vi "Slice Engine.vi"(8 "error in (no error)":errorcluster, 11 "System Parameters":T1={"Vibratome"={"Z Bottom [mm]"=0.0, "Pre Cut Dwell [s]"=1.0, "Blade Frequency [RPM]"=3000, "Slice Speed [mm/s]"=1.0, "Post Cut Dwell [s]"=1.0, "Ramp Time [s]"=0.5, "Start X [mm]"=80.5, "Start Y [mm]"=72.0, "Slice Length [mm]"=25.0, "Slice Axis"=enum."X Axis", "Controller VISA Ref"="COM3"}, "Table Stages"={"X Stage"={"Position"=0.0, "Is.Enabled?"=FALSE, "Is.Connected?"=FALSE, "Device SN"="45875688", "AccelerationMaximum"=50.0, "VelocityMaximum"=50.0, "Acceleration"=20.0, "Velocity"=20.0, "waitTimeout (ms)"=1000000, "Model"=enum."Thorlabs LTS", "Is.Homed?"=FALSE}, "Y Stage"={"Position"=0.0, "Is.Enabled?"=FALSE, "Is.Connected?"=FALSE, "Device SN"="45875512", "AccelerationMaximum"=50.0, "VelocityMaximum"=50.0, "Acceleration"=20.0, "Velocity"=20.0, "waitTimeout (ms)"=1000000, "Model"=enum."Thorlabs LTS", "Is.Homed?"=FALSE}, "Z Stage"={"Position"=0.0, "Is.Enabled?"=FALSE, "Is.Connected?"=FALSE, "Device SN"="49872414", "AccelerationMaximum"=50.0, "VelocityMaximum"=50.0, "Acceleration"=20.0, "Velocity"=20.0, "waitTimeout (ms)"=100000, "Model"=enum."Thorlabs MLJ", "Is.Homed?"=FALSE}}}) -> (0 "error out":errorcluster)   [LabVIEW 2017]
uses:
  Controls/System Parameters.ctl
  Hardware/Table Stage/Controls/Translation Stage Cluster.ctl
  Controls/Translation Stage Types.ctl
  Controls/FGV Actions.ctl
  Controls/Queue Manager Actions.ctl
  Controls/QueueNames.ctl
  Hardware/Table Stage/Controls/Motion Translation Module Control.ctl
  Controls/Set Get Controls.ctl
  Controls/Thorlabs Acq Status.ctl
panel:
  in  "Slice thickness  (mm)":dbl=150.0
  in  "Running":bool
  in  "Last Slice?":bool
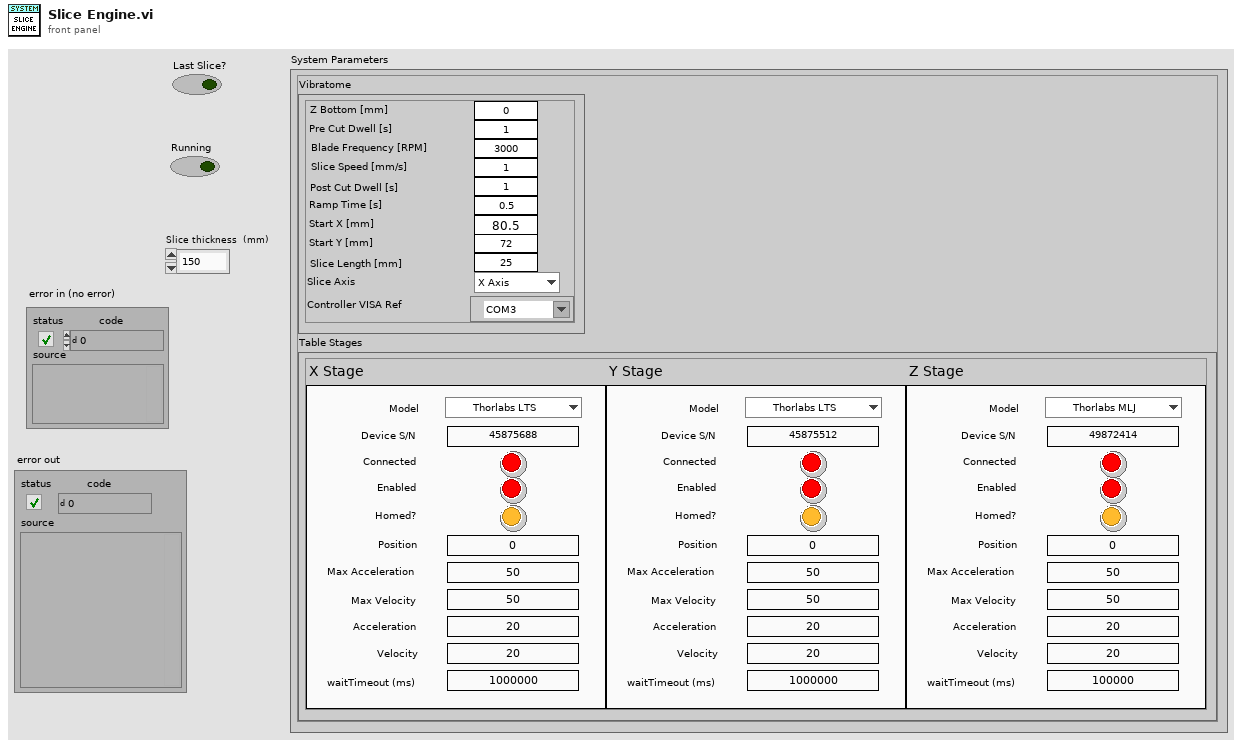
[diagram p1: front panel]
types:
  T1 = typedef "System Parameters.ctl" = cluster{"Vibratome":cluster{"Z Bottom [mm]":dbl, "Pre Cut Dwell [s]":dbl, "Blade Frequency [RPM]":u16, "Slice Speed [mm/s]":dbl, "Post Cut Dwell [s]":dbl, "Ramp Time [s]":dbl, "Start X [mm]":dbl, "Start Y [mm]":dbl, "Slice Length [mm]":dbl, "Slice Axis":enum16{"X Axis", "Y Axis", "Z Axis"}, "Controller VISA Ref":refnum<visa-resource-name>}, "Table Stages":cluster{"X Stage":T2, "Y Stage":T2, "Z Stage":T2}}
  T2 = typedef "Translation Stage Cluster.ctl" = cluster{"Position":dbl, "Is.Enabled?":bool, "Is.Connected?":bool, "Device SN":string, "AccelerationMaximum":dbl, "VelocityMaximum":dbl, "Acceleration":dbl, "Velocity":dbl, "waitTimeout (ms)":i32, "Model":T3, "Is.Homed?":bool}
  T3 = typedef "Translation Stage Types.ctl" = enum16{"None", "Thorlabs LTS", "Thorlabs MLJ"}
  T4 = typedef "FGV Actions.ctl" = enum16{"Init", "Set", "Get", "Clear"}
  T5 = typedef "QueueNames.ctl" = enum16{"Main GUI", "Main Scan Processor", "Main Display", "Main Table Stage GUI", "Main Table Stage Proc.", "Scan Engine", "Vibratome GUI", "Vibratome Processor", "Slice Engine"}
  T6 = typedef "Queue Manager Actions.ctl" = enum16{"Init", "Enqueue", "Enqueue All", "Preview Queue", "Dequeue", "Get Status", "Flush Queue", "Flush All Queues", "Release All Queues", "Release Queue", "Enqueue at Opposite End"}
  T7 = typedef "Set Get Controls.ctl" = enum16{"Set", "Get"}
  T8 = typedef "Motion Translation Module Control.ctl" = enum16{"Init", "Home", "Status", "Velocity/Accel", "Position", "Jog", "Stop", "Uninit", "Enable", "Disable"}
  T9 = enum16{"Set Configuration", "Get Configuration", "Enable Motor", "Disable Motor", "Get Status", "Open Session", "Close Session", "Set Limits", "Get Limits"}
  T10 = cluster{"Source for Velocity":enum16{"Interface", "Voltage (AI)", "PWM (AI)", "Current Target (AI)", "Current Target w/ Preset (AI)"}, "Mode":enum16{"Continuous", "Stepper Motor", "Analog Position Ctrl", "Encoder"}, "Target Velocity [RPM]":i16}
  T11 = typedef "Thorlabs Acq Status.ctl" = enum16{"Idle", "Image", "Translate"}
  T12 = typedef "MessagePacket.ctl" = cluster{"Message":string, "Parameter":variant}
  T13 = cluster{"X Stage":T2, "Y Stage":T2, "Z Stage":T2}
  T14 = cluster{"Z Bottom [mm]":dbl, "Pre Cut Dwell [s]":dbl, "Blade Frequency [RPM]":u16, "Slice Speed [mm/s]":dbl, "Post Cut Dwell [s]":dbl, "Ramp Time [s]":dbl, "Start X [mm]":dbl, "Start Y [mm]":dbl, "Slice Length [mm]":dbl, "Slice Axis":enum16{"X Axis", "Y Axis", "Z Axis"}, "Controller VISA Ref":refnum<visa-resource-name>}
  T15 = enum16{"Left Button", "Center Button", "Right Button", "Window Close"}
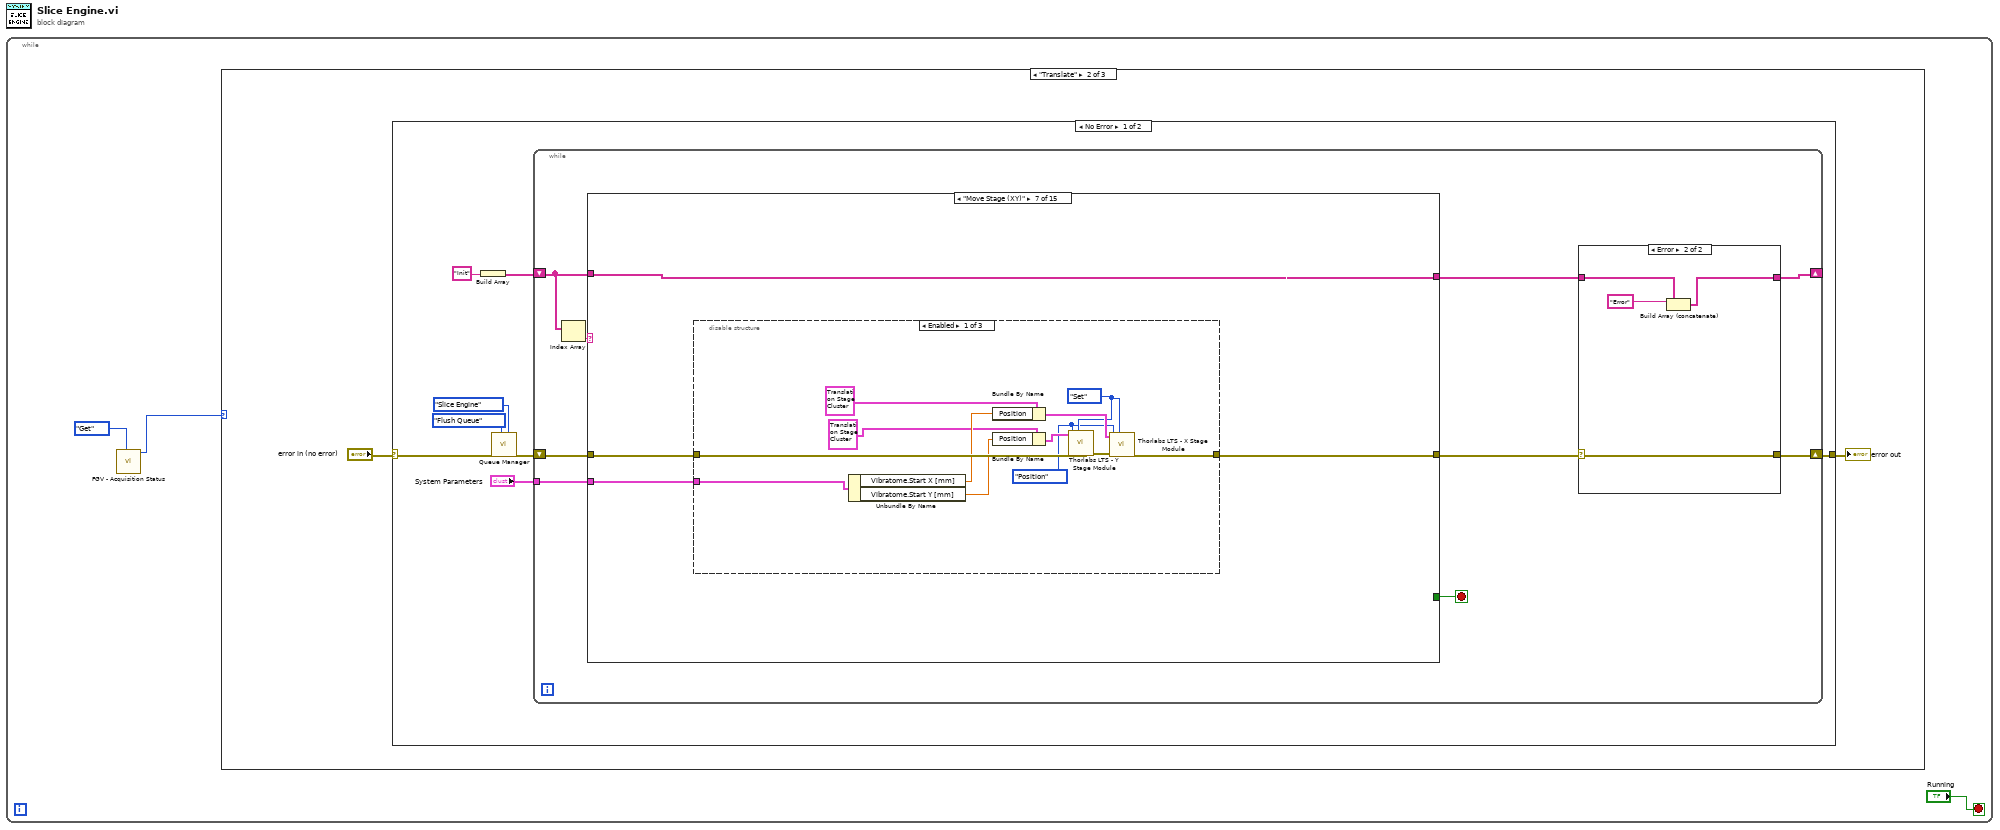
[diagram p0: block diagram]
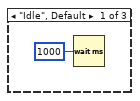
[diagram p2: hidden frame]
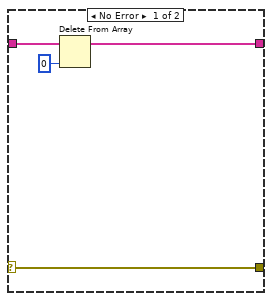
[diagram p3: hidden frame]
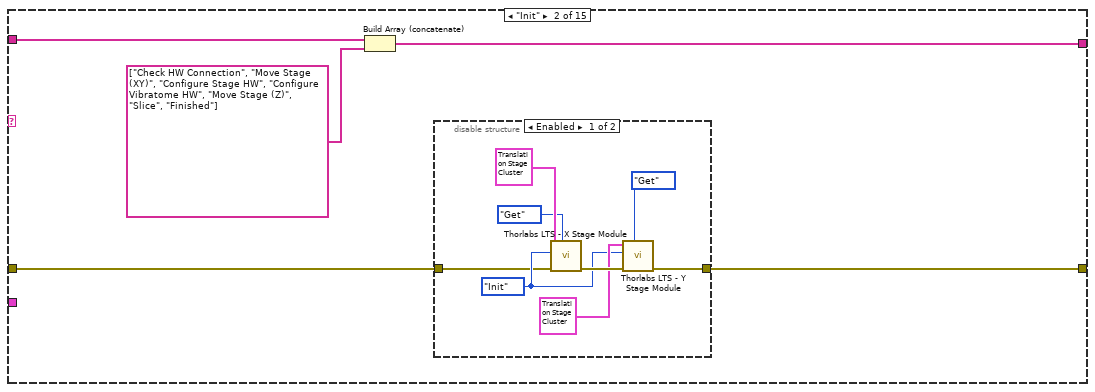
[diagram p5: hidden frame]
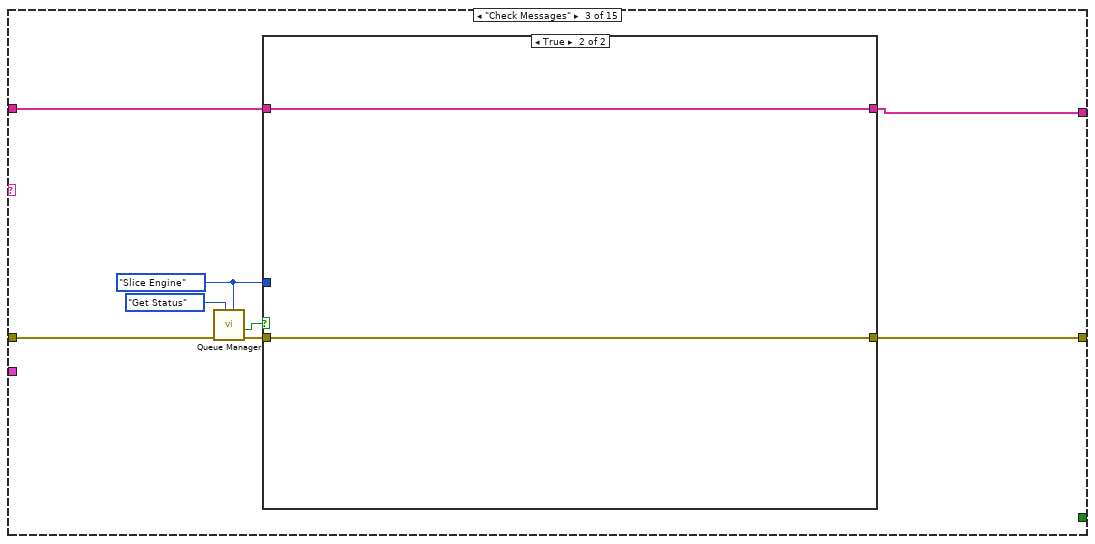
[diagram p7: hidden frame]
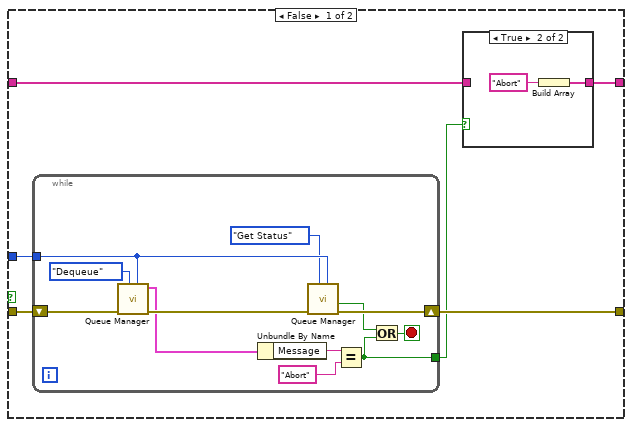
[diagram p8: hidden frame]
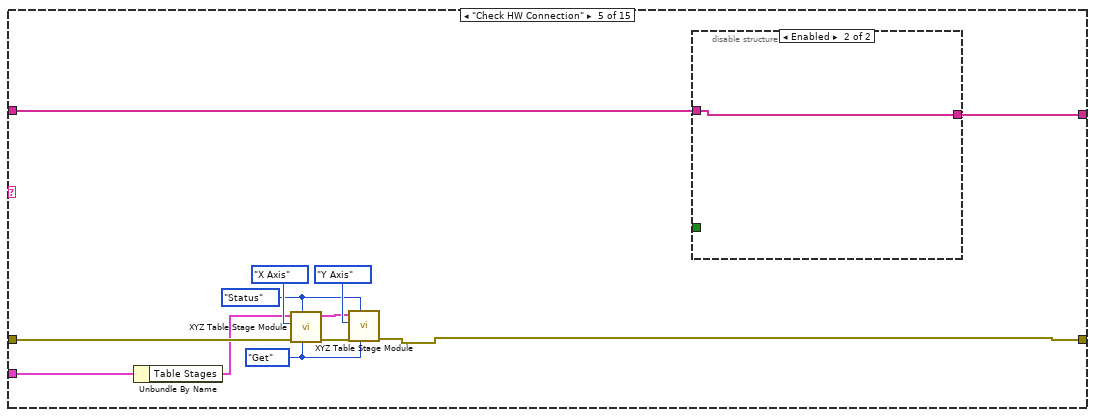
[diagram p11: hidden frame]
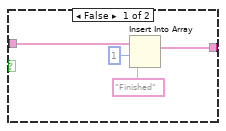
[diagram p13: hidden frame]
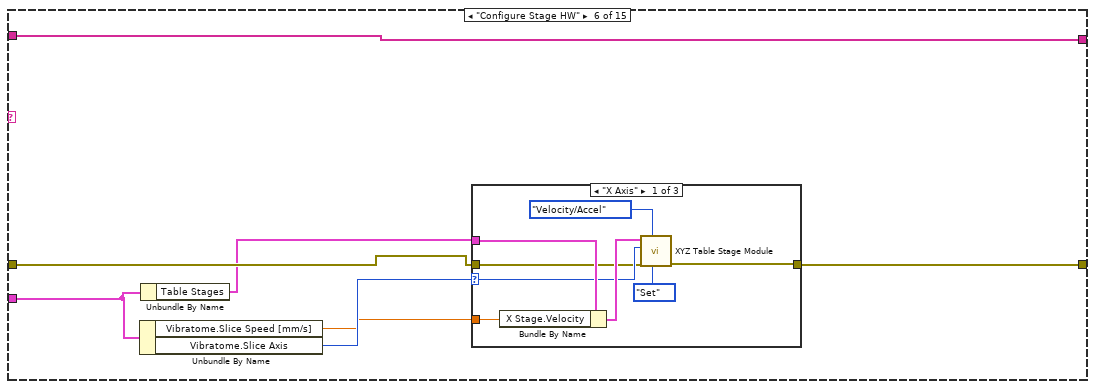
[diagram p14: hidden frame]
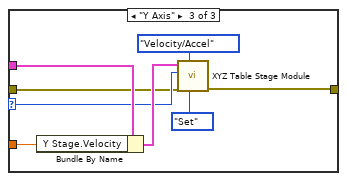
[diagram p16: hidden frame]
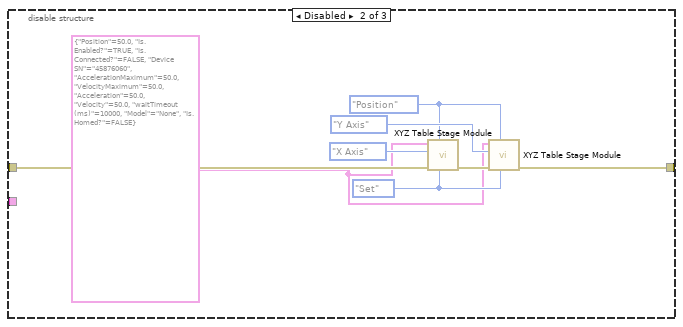
[diagram p17: hidden frame]
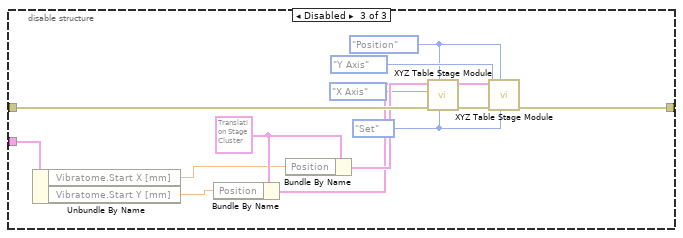
[diagram p18: hidden frame]
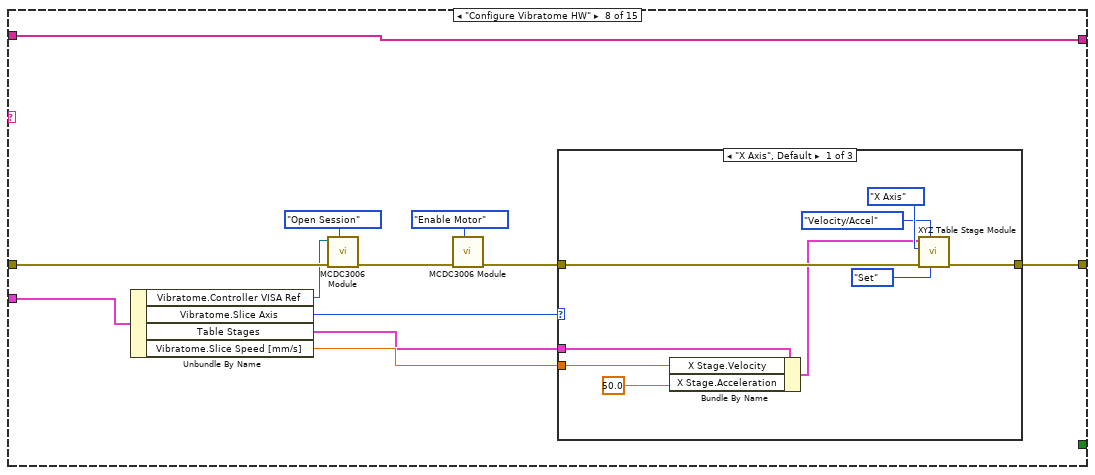
[diagram p19: hidden frame]
diagram:
  n1 = while {
    stop <- "Running" stop-if-true
    n2 = call "FGV - Acquisition Status.vi"("Actions"=FGV_Actions."Get") -> ("Action [Out]"=w2:T11)  [unwired: 9 in, 1 out]
    n3 = case shown="\"Translate\"" w2 {
      frame "Idle", Default {
        n4 = Wait (ms)(milliseconds to wait=u32 1000) -> ()  [unwired: 1 out]
      }
      frame "Translate" {
        n5 = case shown="No Error" "error in (no error)" {
          selector: "error in (no error)" -> [w7 w420]
          tunnel: [w9 w420] -> w5
          frame No Error {
            n6 = Build Array("Init") -> (w10:string[])
            n7 = call "Queue Manager.vi"("Queue Name"=QueueNames."Slice Engine", "Action"=Queue_Manager_Actions."Flush Queue", "Error In"=w7) -> ("Error Out"=w13:errorcluster)  [unwired: 4 in, 4 out]
            n8 = while {
              shift-right: [w17] -> _
              shift-left: w10 -> [w16]
              shift-right: [w19] -> w9
              shift-left: w13 -> [w23]
              tunnel: "System Parameters" -> [w15]
              stop <- w21 stop-if-true
              n9 = Index Array(array=w16) -> (element=w22:string)  [unwired: 1 in]
              n10 = case shown="\"Move Stage (XY)\"" w22 {
                tunnel: w23 -> [w32 w35 w55 w79 w92 w103 w129 w172 w199 w212 w276 w290 w294 w323 w391]
                tunnel: w16 -> [w33 w38 w49 w80 w82 w108 w126 w174 w210 w211 w279 w287 w292 w324 w402]
                tunnel: [w33 w37 w48 w80 w83 w108 w126 w174 w210 w211 w278 w288 w291 w324 w402] -> w18
                tunnel: [_ _ _ _ _ _ _ _ _ _ _ _ _ _ TRUE] -> w21
                tunnel: [w32 w34 w50 w79 w81 w104 w128 w166 w203 w213 w276 w290 w295 w321 w398] -> w20
                tunnel: w15 -> [_ _ _ _ w91 w107 w127 w173 w209 w214 _ _ _ w322 w394]
                frame "Unknown", Default {
                }
                frame "Init" {
                  n11 = Build Array (concatenate)(w38, string[] ["Check HW Connection", "Move Stage (XY)", "Configure Stage HW", "Configure Vibratome HW", "Move Stage (Z)", "Slice", "Finished"]) -> (w37:string[])
                  n12 = disable-structure shown="Enabled" {
                    disable-tunnel: w35 -> [w40 w47]
                    disable-tunnel: [w39 w47] -> w34
                    frame Enabled {
                      w43 = Motion_Translation_Module_Control."Init" ("Action")
                      n13 = call "Thorlabs LTS - X Stage Module.vi"("Set/Get"=Set_Get_Controls."Get", "Error In"=w40, "Action"=w43, "Cluster In"=T2 {"Position"=0.0, "Is.Enabled?"=TRUE, "Is.Connected?"=FALSE, "Device SN"="45875688", "AccelerationMaximum"=0.0, "VelocityMaximum"=0.0, "Acceleration"=0.0, "Velocity"=0.0, "waitTimeout (ms)"=10000, "Model"=enum."None", "Is.Homed?"=FALSE}) -> ("Error Out"=w46:errorcluster)  [unwired: 6 in, 1 out]
                      n14 = call "Thorlabs LTS - Y Stage Module.vi"("Set/Get"=Set_Get_Controls."Get", "Error In"=w46, "Action"=w43, "Cluster In"=T2 {"Position"=0.0, "Is.Enabled?"=TRUE, "Is.Connected?"=FALSE, "Device SN"="45875512", "AccelerationMaximum"=0.0, "VelocityMaximum"=0.0, "Acceleration"=0.0, "Velocity"=0.0, "waitTimeout (ms)"=10000, "Model"=enum."None", "Is.Homed?"=FALSE}) -> ("Error Out"=w39:errorcluster)  [unwired: 6 in, 1 out]
                    }
                    frame Disabled {
                    }
                  }
                }
                frame "Check Messages" {
                  w51 = QueueNames."Slice Engine" ("Queue Name")
                  n15 = call "Queue Manager.vi"("Queue Name"=w51, "Action"=Queue_Manager_Actions."Get Status", "Error In"=w55) -> ("Error Out"=w52:errorcluster, "Empty?"=w53:bool)  [unwired: 4 in, 3 out]
                  n16 = case shown="True" w53 {
                    tunnel: w52 -> [w61 w77]
                    tunnel: w51 -> [w60 _]
                    tunnel: [w59 w77] -> w50
                    tunnel: w49 -> [w57 w78]
                    tunnel: [w56 w78] -> w48
                    frame False {
                      n17 = while {
                        tunnel: w60 -> [w72]
                        shift-right: [w73] -> w59
                        shift-left: w61 -> [w76]
                        tunnel: [w65] -> w58
                        stop <- w66 stop-if-true
                        n18 = call "Queue Manager.vi"("Queue Name"=w72, "Action"=Queue_Manager_Actions."Dequeue", "Error In"=w76) -> ("Error Out"=w74:errorcluster, "Message Packet [Out]"=w70:T12)  [unwired: 4 in, 3 out]
                        n19 = Unbundle By Name(w70) -> ("Message"=w69:string)
                        n20 = call "Queue Manager.vi"("Queue Name"=w72, "Action"=Queue_Manager_Actions."Get Status", "Error In"=w74) -> ("Error Out"=w73:errorcluster, "Empty?"=w67:bool)  [unwired: 4 in, 3 out]
                        n21 = Equal?(x=w69, y="Abort") -> (x = y?=w65:bool)
                        n22 = Or(x=w67, y=w65) -> (x .or. y?=w66:bool)
                      }
                      n23 = case shown="True" w58 {
                        tunnel: w57 -> [w62 _]
                        tunnel: [w62 w63] -> w56
                        frame False {
                        }
                        frame True {
                          n24 = Build Array("Abort") -> (w63:string[])
                        }
                      }
                    }
                    frame True {
                    }
                  }
                }
                frame "Load Parameters" {
                }
                frame "Check HW Connection" {
                  w86 = Set_Get_Controls."Get" ("Set/Get")
                  w87 = Motion_Translation_Module_Control."Status" ("Action")
                  n25 = Unbundle By Name(w91) -> ("Table Stages"=w85:T13)
                  n26 = call "XYZ Table Stage Module.vi"("Set/Get"=w86, "Action"=w87, "Error In"=w92, "Axis"=enum16{"X Axis", "Y Axis", "Z Axis"}."X Axis", "Table Stages"=w85) -> ("Error Out"=w90:errorcluster, "Table Stages Out"=w84:T13)  [unwired: 5 in]
                  n27 = call "XYZ Table Stage Module.vi"("Set/Get"=w86, "Action"=w87, "Error In"=w90, "Axis"=enum16{"X Axis", "Y Axis", "Z Axis"}."Y Axis", "Table Stages"=w84) -> ("Error Out"=w81:errorcluster)  [unwired: 5 in, 1 out]
                  n28 = disable-structure shown="Enabled" {
                    disable-tunnel: [w95 w101] -> w83
                    disable-tunnel: w82 -> [w94 w101]
                    disable-tunnel: _ -> [w93 _]
                    frame Disabled {
                      n29 = case "Checks Stage Status OK" shown="True" w93 {
                        tunnel: [w99 w100] -> w95
                        tunnel: w94 -> [w98 w100]
                        frame False {
                          n30 = Insert Into Array(array=w98, index=1, new element="Finished" ("new element/subarray")) -> (w99:string[])
                        }
                        frame True {
                        }
                      }
                    }
                    frame Enabled {
                    }
                  }
                }
                frame "Configure Stage HW" {
                  n31 = Unbundle By Name(w107) -> ("Vibratome.Slice Speed [mm/s]"=w105:dbl, "Vibratome.Slice Axis"=w106:enum16{"X Axis", "Y Axis", "Z Axis"})
                  n32 = Unbundle By Name(w107) -> ("Table Stages"=w102:T13)
                  n33 = case shown="\"X Axis\"" w106 {
                    selector: w106 -> [w113 _ w122]
                    tunnel: w105 -> [w116 _ w125]
                    tunnel: w102 -> [w115 _ w124]
                    tunnel: w103 -> [w112 w117 w121]
                    tunnel: [w111 w117 w120] -> w104
                    frame "X Axis" {
                      n34 = Bundle By Name(cluster=w115, "X Stage.Velocity"=w116) -> (w114:T13)
                      n35 = call "XYZ Table Stage Module.vi"("Set/Get"=Set_Get_Controls."Set", "Action"=Motion_Translation_Module_Control."Velocity/Accel", "Error In"=w112, "Axis"=w113, "Table Stages"=w114) -> ("Error Out"=w111:errorcluster)  [unwired: 5 in, 1 out]
                    }
                    frame "Z Axis" {
                    }
                    frame "Y Axis" {
                      n36 = Bundle By Name(cluster=w124, "Y Stage.Velocity"=w125) -> (w123:T13)
                      n37 = call "XYZ Table Stage Module.vi"("Set/Get"=Set_Get_Controls."Set", "Action"=Motion_Translation_Module_Control."Velocity/Accel", "Error In"=w121, "Axis"=w122, "Table Stages"=w123) -> ("Error Out"=w120:errorcluster)  [unwired: 5 in, 1 out]
                    }
                  }
                }
                frame "Move Stage (XY)" {
                  n38 = disable-structure shown="Enabled" {
                    disable-tunnel: w129 -> [w141 w147 w160]
                    disable-tunnel: [w130 w148 w161] -> w128
                    disable-tunnel: w127 -> [w137 _ w159]
                    frame Enabled {
                      w133 = Motion_Translation_Module_Control."Position" ("Action")
                      w134 = Set_Get_Controls."Set" ("Set/Get")
                      n39 = Unbundle By Name(w137) -> ("Vibratome.Start X [mm]"=w136:dbl, "Vibratome.Start Y [mm]"=w135:dbl)
                      n40 = Bundle By Name(cluster=T2 {"Position"=0.0, "Is.Enabled?"=TRUE, "Is.Connected?"=FALSE, "Device SN"="45875688", "AccelerationMaximum"=50.0, "VelocityMaximum"=50.0, "Acceleration"=50.0, "Velocity"=50.0, "waitTimeout (ms)"=10000000, "Model"=enum."Thorlabs LTS", "Is.Homed?"=FALSE} ("Cluster In"), "Position"=w136) -> (w140:T2)
                      n41 = Bundle By Name(cluster=T2 {"Position"=0.0, "Is.Enabled?"=TRUE, "Is.Connected?"=FALSE, "Device SN"="45875512", "AccelerationMaximum"=50.0, "VelocityMaximum"=50.0, "Acceleration"=50.0, "Velocity"=50.0, "waitTimeout (ms)"=10000000, "Model"=enum."Thorlabs LTS", "Is.Homed?"=FALSE} ("Cluster In"), "Position"=w135) -> (w138:T2)
                      n42 = call "Thorlabs LTS - Y Stage Module.vi"("Set/Get"=w134, "Error In"=w141, "Action"=w133, "Cluster In"=w138) -> ("Error Out"=w131:errorcluster)  [unwired: 6 in, 1 out]
                      n43 = call "Thorlabs LTS - X Stage Module.vi"("Set/Get"=w134, "Error In"=w131, "Action"=w133, "Cluster In"=w140) -> ("Error Out"=w130:errorcluster)  [unwired: 6 in, 1 out]
                    }
                    frame Disabled {
                      w143 = Set_Get_Controls."Set" ("Set/Get")
                      w144 = Motion_Translation_Module_Control."Position" ("Action")
                      w142 = T2 {"Position"=50.0, "Is.Enabled?"=TRUE, "Is.Connected?"=FALSE, "Device SN"="45876060", "AccelerationMaximum"=50.0, "VelocityMaximum"=50.0, "Acceleration"=50.0, "Velocity"=50.0, "waitTimeout (ms)"=10000, "Model"=enum."None", "Is.Homed?"=FALSE} ("Cluster In")
                      n44 = call "XYZ Table Stage Module.vi"("Set/Get"=w143, "Action"=w144, "Error In"=w147, "Axis"=enum16{"X Axis", "Y Axis", "Z Axis"}."X Axis", "Table Stages"=w142) -> ("Error Out"=w149:errorcluster)  [unwired: 5 in, 1 out]
                      n45 = call "XYZ Table Stage Module.vi"("Set/Get"=w143, "Action"=w144, "Error In"=w149, "Axis"=enum16{"X Axis", "Y Axis", "Z Axis"}."Y Axis", "Table Stages"=w142) -> ("Error Out"=w148:errorcluster)  [unwired: 5 in, 1 out]
                    }
                    frame Disabled {
                      w150 = Set_Get_Controls."Set" ("Set/Get")
                      w151 = Motion_Translation_Module_Control."Position" ("Action")
                      w158 = T2 {"Position"=0.0, "Is.Enabled?"=TRUE, "Is.Connected?"=FALSE, "Device SN"="45876060", "AccelerationMaximum"=50.0, "VelocityMaximum"=50.0, "Acceleration"=50.0, "Velocity"=50.0, "waitTimeout (ms)"=10000, "Model"=enum."None", "Is.Homed?"=FALSE} ("Cluster In")
                      n46 = Unbundle By Name(w159) -> ("Vibratome.Start X [mm]"=w157:dbl, "Vibratome.Start Y [mm]"=w156:dbl)
                      n47 = Bundle By Name(cluster=w158, "Position"=w156) -> (w154:T2)
                      n48 = Bundle By Name(cluster=w158, "Position"=w157) -> (w155:T2)
                      n49 = call "XYZ Table Stage Module.vi"("Set/Get"=w150, "Action"=w151, "Error In"=w160, "Axis"=enum16{"X Axis", "Y Axis", "Z Axis"}."X Axis", "Table Stages"=w155) -> ("Error Out"=w162:errorcluster)  [unwired: 5 in, 1 out]
                      n50 = call "XYZ Table Stage Module.vi"("Set/Get"=w150, "Action"=w151, "Error In"=w162, "Axis"=enum16{"X Axis", "Y Axis", "Z Axis"}."Y Axis", "Table Stages"=w154) -> ("Error Out"=w161:errorcluster)  [unwired: 5 in, 1 out]
                    }
                  }
                }
                frame "Configure Vibratome HW" {
                  n51 = Unbundle By Name(w173) -> ("Vibratome.Controller VISA Ref"=w170:refnum<visa-resource-name>, "Vibratome.Slice Axis"=w165:enum16{"X Axis", "Y Axis", "Z Axis"}, "Table Stages"=w163:T13, "Vibratome.Slice Speed [mm/s]"=w164:dbl)
                  n52 = call "MCDC3006 Module.vi"("Actions"=T9."Open Session", "Error In"=w172, "VISA resource name"=w170) -> ("Error Out"=w168:errorcluster)  [unwired: 4 in, 4 out]
                  n53 = call "MCDC3006 Module.vi"("Actions"=T9."Enable Motor", "Error In"=w168) -> ("Error Out"=w167:errorcluster)  [unwired: 5 in, 4 out]
                  n54 = case shown="\"X Axis\", Default" w165 {
                    tunnel: [w183 w184 w193] -> w166
                    tunnel: w167 -> [w178 w184 w189]
                    tunnel: w164 -> [w179 _ w188]
                    tunnel: w163 -> [w176 _ w187]
                    frame "X Axis", Default {
                      n55 = Bundle By Name(cluster=w176, "X Stage.Velocity"=w179, "X Stage.Acceleration"=50.0 ("Acceleration")) -> (w175:T13)
                      n56 = call "XYZ Table Stage Module.vi"("Set/Get"=Set_Get_Controls."Set", "Action"=Motion_Translation_Module_Control."Velocity/Accel", "Error In"=w178, "Axis"=enum16{"X Axis", "Y Axis", "Z Axis"}."X Axis", "Table Stages"=w175) -> ("Error Out"=w183:errorcluster)  [unwired: 5 in, 1 out]
                    }
                    frame "Z Axis" {
                    }
                    frame "Y Axis" {
                      n57 = Bundle By Name(cluster=w187, "Y Stage.Velocity"=w188, "Y Stage.Acceleration"=50.0 ("Acceleration")) -> (w185:T13)
                      n58 = call "XYZ Table Stage Module.vi"("Set/Get"=Set_Get_Controls."Set", "Action"=Motion_Translation_Module_Control."Velocity/Accel", "Error In"=w189, "Axis"=enum16{"X Axis", "Y Axis", "Z Axis"}."Y Axis", "Table Stages"=w185) -> ("Error Out"=w193:errorcluster)  [unwired: 5 in, 1 out]
                    }
                  }
                }
                frame "Move Stage (Z)" {
                  n59 = Unbundle By Name(w209) -> ("Table Stages.Z Stage"=w198:T2)
                  n60 = call "Thorlabs MLJ - Z Stage Module.vi"("Set/Get"=Set_Get_Controls."Get", "Error In"=w199, "Action"=Motion_Translation_Module_Control."Position", "Cluster In"=w198) -> ("Error Out"=w205:errorcluster, "Cluster Out"=w201:T2)  [unwired: 6 in]
                  n61 = Unbundle By Name(w201) -> ("Position"=w197:dbl)
                  n62 = Divide(x="Slice thickness  (mm)", y=1000.0) -> (x/y=w196:dbl)
                  n63 = Add(x=w197, y=w196) -> (x+y=w202:dbl)
                  n64 = Bundle By Name(cluster=w201, "Position"=w202) -> (w200:T2)
                  n65 = call "Thorlabs MLJ - Z Stage Module.vi"("Set/Get"=Set_Get_Controls."Set", "Error In"=w205, "Action"=Motion_Translation_Module_Control."Position", "Cluster In"=w200) -> ("Error Out"=w203:errorcluster)  [unwired: 6 in, 1 out]
                }
                frame "Slice" {
                  n66 = disable-structure shown="Enabled" {
                    disable-tunnel: w214 -> [w227 w273]
                    disable-tunnel: [w217 w274] -> w213
                    disable-tunnel: w212 -> [w216 w275]
                    frame Enabled {
                      n67 = Unbundle By Name(w227) -> ("Vibratome.Blade Frequency [RPM]"=w221:u16, "Vibratome.Slice Axis"=w226:enum16{"X Axis", "Y Axis", "Z Axis"}, "Vibratome.Slice Length [mm]"=w225:dbl, "Vibratome.Post Cut Dwell [s]"=w219:dbl, "Vibratome.Pre Cut Dwell [s]"=w218:dbl, "Table Stages.X Stage"=w215:T2)
                      n68 = Bundle By Name(cluster=T10 {"Source for Velocity"=enum."Interface", "Mode"=enum."Continuous", "Target Velocity [RPM]"=0} ("Configuration [In]"), "Target Velocity [RPM]"=w221) -> (w220:T10)
                      n69 = call "MCDC3006 Module.vi"("Actions"=T9."Set Configuration", "Error In"=w216, "Configuration [In]"=w220) -> ("Error Out"=w224:errorcluster)  [unwired: 4 in, 4 out]
                      n70 = case shown="\"X Axis\"" w226 {
                        tunnel: w224 -> [w253 w254 w271]
                        tunnel: [w241 w254 w258] -> w217
                        tunnel: w225 -> [w247 _ w265]
                        tunnel: w219 -> [w244 _ w261]
                        tunnel: w218 -> [w236 _ _]
                        tunnel: w215 -> [w231 _ _]
                        frame "X Axis" {
                          w238 = Motion_Translation_Module_Control."Position" ("Action")
                          n71 = expression code="x*1000"(w236) -> (w235:dbl)
                          n72 = To Unsigned Long Integer(number=w235) -> (unsigned 32bit integer=w234:u32)
                          n73 = call "Inline Wait.vi"("Error In"=w253, "milliseconds to wait"=w234) -> ("Error Out"=w237:errorcluster)  [unwired: 9 in]
                          n74 = expression code="x*1000"(w244) -> (w243:dbl)
                          n75 = call "Thorlabs LTS - X Stage Module.vi"("Set/Get"=Set_Get_Controls."Get", "Error In"=w237, "Action"=w238, "Cluster In"=w231) -> ("Error Out"=w252:errorcluster, "Cluster Out"=w239:T2)  [unwired: 6 in]
                          n76 = To Unsigned Long Integer(number=w243) -> (unsigned 32bit integer=w242:u32)
                          n77 = Unbundle By Name(w239) -> ("Position"=w248:dbl)
                          n78 = Add(x=w248, y=w247) -> (x+y=w246:dbl)
                          n79 = Bundle By Name(cluster=w239, "Position"=w246) -> (w245:T2)
                          n80 = call "Thorlabs LTS - X Stage Module.vi"("Set/Get"=Set_Get_Controls."Set", "Error In"=w252, "Action"=w238, "Cluster In"=w245) -> ("Error Out"=w250:errorcluster)  [unwired: 6 in, 1 out]
                          n81 = call "Inline Wait.vi"("Error In"=w250, "milliseconds to wait"=w242) -> ("Error Out"=w233:errorcluster)  [unwired: 9 in]
                          n82 = call "MCDC3006 Module.vi"("Actions"=T9."Disable Motor", "Error In"=w233) -> ("Error Out"=w229:errorcluster)  [unwired: 5 in, 4 out]
                          n83 = call "MCDC3006 Module.vi"("Actions"=T9."Close Session", "Error In"=w229) -> ("Error Out"=w228:errorcluster)  [unwired: 5 in, 4 out]
                          n84 = call "Thorlabs LTS - X Stage Module.vi"("Set/Get"=Set_Get_Controls."Set", "Error In"=w228, "Action"=w238, "Cluster In"=w239) -> ("Error Out"=w241:errorcluster)  [unwired: 6 in, 1 out]
                        }
                        frame "Z Axis" {
                        }
                        frame "Y Axis" {
                          w255 = Motion_Translation_Module_Control."Position" ("Action")
                          n85 = expression code="x*1000"(w261) -> (w260:dbl)
                          n86 = call "Thorlabs LTS - Y Stage Module.vi"("Set/Get"=Set_Get_Controls."Get", "Error In"=w271, "Action"=w255) -> ("Error Out"=w270:errorcluster, "Cluster Out"=w256:T2)  [unwired: 7 in]
                          n87 = To Unsigned Long Integer(number=w260) -> (unsigned 32bit integer=w259:u32)
                          n88 = Unbundle By Name(w256) -> ("Position"=w266:dbl)
                          n89 = Add(x=w266, y=w265) -> (x+y=w264:dbl)
                          n90 = Bundle By Name(cluster=w256, "Position"=w264) -> (w263:T2)
                          n91 = call "Thorlabs LTS - Y Stage Module.vi"("Set/Get"=Set_Get_Controls."Set", "Error In"=w270, "Action"=w255, "Cluster In"=w263) -> ("Error Out"=w268:errorcluster)  [unwired: 6 in, 1 out]
                          n92 = call "Inline Wait.vi"("Error In"=w268, "milliseconds to wait"=w259) -> ("Error Out"=w262:errorcluster)  [unwired: 9 in]
                          n93 = call "Thorlabs LTS - Y Stage Module.vi"("Set/Get"=Set_Get_Controls."Set", "Error In"=w262, "Action"=w255, "Cluster In"=w256) -> ("Error Out"=w258:errorcluster)  [unwired: 6 in, 1 out]
                        }
                      }
                    }
                    frame Disabled {
                      n94 = Unbundle By Name(w273) -> ("Vibratome"=w272:T14)
                      n95 = call "Slice Module.vi"("Error In"=w275, "Vibratome"=w272) -> ("Error Out"=w274:errorcluster)  [unwired: 7 in, 2 out]
                    }
                  }
                }
                frame "Next Slice" {
                  n96 = case shown="False" "Last Slice?" {
                    tunnel: w279 -> [w283 w284]
                    tunnel: [w282 w284] -> w278
                    frame False {
                      n97 = Insert Into Array(array=w283, index=1, new element=string[] ["Move Stage (Z)", "Slice", "Next Slice"]) -> (w282:string[])
                    }
                    frame True {
                    }
                  }
                }
                frame "Abort" {
                  n98 = Insert Into Array(array=w287, index=1, new element #1="Uninit", new element #2="Finished") -> (w288:string[])
                }
                frame "Error" {
                  n99 = control-ref of="This VI"() -> (w305:refnum<vi>)
                  n100 = property class="VI"(reference=w305) -> ("Name"=w308:string, "Callers"=w310:string[])  [unwired: 1 in, 2 out]
                  n101 = Unbundle(w294) -> ("code"=w304:i32, "source"=w303:string)  [unwired: 1 out]
                  n102 = Array To Spreadsheet String(delimiter (Tab)=">", array=w310, 3:"%s" ("format string")) -> (spreadsheet string=w309:string)
                  n103 = Format Into String(format string="VI Name: %s\nCallers: %s\nError Code: %d\nError Message: %s", initial string="The following error occurred:\n" ("message"), w308, w309, w304, w303) -> (resulting string=w302:string, error out=w296:errorcluster)  [unwired: 1 in]
                  n104 = call <vilib>:"Clear Errors.vi"("error in (no error)"=w296) -> ()  [unwired: 5 in, 2 out]
                  n105 = call <vilib>:"Three Button Dialog.vi"("Allow user to close window? (TRUE)"=FALSE, "Window Title (\"\")"="Error" ("Window Title (\"\")"), "Right Button Text (\"Cancel\")"="Abort" ("Right Button Text (\"Cancel\")"), "Center Button Text (\"No\")"="Retry" ("Center Button Text (\"No\")"), "Left Button Text (\"Yes\")"="Continue" ("Left Button Text (\"Yes\")"), "message"=w302) -> ("Which Button?"=w293:T15)  [unwired: 5 in]
                  n106 = case shown="\"Right Button\"" w293 {
                    tunnel: w292 -> [w315 w319 w320]
                    tunnel: [w314 w318 w320] -> w291
                    frame "Left Button", Default {
                      # "Continue"
                      n107 = Delete From Array(array=w315, index=0) -> (array with subset deleted=w314:string[])  [unwired: 1 in, 1 out]
                    }
                    frame "Right Button" {
                      # "Abort"
                      n108 = Insert Into Array(array=w319, index=1, new element="Abort") -> (w318:string[])
                    }
                    frame "Center Button" {
                      # "Retry"
                    }
                  }
                  n109 = call <vilib>:"Clear Errors.vi"("error in (no error)"=w294) -> ("error out"=w295:errorcluster)  [unwired: 5 in, 1 out]
                }
                frame "Uninit" {
                  n110 = disable-structure shown="Enabled" {
                    disable-tunnel: w323 -> [w328 w389]
                    disable-tunnel: w322 -> [w327 _]
                    disable-tunnel: [w326 w382] -> w321
                    frame Enabled {
                      n111 = for {
                        N: 4 -> [_]
                        tunnel: [w334] -> w329 mode=indexing
                        tunnel: Motion_Translation_Module_Control."Uninit" ("Action") -> [w333]
                        tunnel: w328 -> [w332]
                        tunnel: w327 -> [w331]
                        i -> [w335]
                        n112 = case shown="3" w335 {
                          tunnel: [w341 w353 w367 w376] -> w334
                          tunnel: w332 -> [w340 w352 w366 w376]
                          tunnel: w333 -> [w339 w351 w365 _]
                          tunnel: w331 -> [w338 w350 w364 _]
                          frame 0, Default {
                            # "X Stage"
                            n113 = Unbundle By Name(w338) -> ("Table Stages.X Stage.Model"=w337:T3, "Table Stages.X Stage"=w336:T2)
                            n114 = case shown="\"Thorlabs LTS\"" w337 {
                              tunnel: [w342 w347] -> w341
                              tunnel: w340 -> [w342 w346]
                              tunnel: w339 -> [_ w345]
                              tunnel: w336 -> [_ w343]
                              frame "None", Default {
                              }
                              frame "Thorlabs LTS" {
                                n115 = call "Thorlabs LTS - X Stage Module.vi"("Set/Get"=Set_Get_Controls."Set", "Error In"=w346, "Action"=w345, "Cluster In"=w343) -> ("Error Out"=w347:errorcluster)  [unwired: 6 in, 1 out]
                              }
                            }
                          }
                          frame 1 {
                            # "Y Stage"
                            n116 = Unbundle By Name(w350) -> ("Table Stages.Y Stage.Model"=w349:T3, "Table Stages.Y Stage.Device SN"=w348:string)
                            n117 = case shown="\"Thorlabs LTS\"" w349 {
                              tunnel: [w354 w361] -> w353
                              tunnel: w352 -> [w354 w360]
                              tunnel: w351 -> [_ w359]
                              tunnel: w348 -> [_ w357]
                              frame "None", Default {
                              }
                              frame "Thorlabs LTS" {
                                n118 = Bundle By Name(cluster=T2 {"Position"=0.0, "Is.Enabled?"=TRUE, "Is.Connected?"=FALSE, "Device SN"="45876539", "AccelerationMaximum"=0.0, "VelocityMaximum"=0.0, "Acceleration"=0.0, "Velocity"=0.0, "waitTimeout (ms)"=0, "Model"=enum."Thorlabs LTS", "Is.Homed?"=FALSE} ("Cluster In"), "Device SN"=w357) -> (w356:T2)
                                n119 = call "Thorlabs LTS - Y Stage Module.vi"("Set/Get"=Set_Get_Controls."Set", "Error In"=w360, "Action"=w359, "Cluster In"=w356) -> ("Error Out"=w361:errorcluster)  [unwired: 6 in, 1 out]
                              }
                            }
                          }
                          frame 2 {
                            # "Z Stage"
                            n120 = Unbundle By Name(w364) -> ("Table Stages.Z Stage.Model"=w363:T3, "Table Stages.Z Stage.Device SN"=w362:string)
                            n121 = case shown="\"Thorlabs MLJ\"" w363 {
                              tunnel: [w368 w375] -> w367
                              tunnel: w366 -> [w368 w374]
                              tunnel: w365 -> [_ w373]
                              tunnel: w362 -> [_ w371]
                              frame "None", Default {
                              }
                              frame "Thorlabs MLJ" {
                                n122 = Bundle By Name(cluster=T2 {"Position"=0.0, "Is.Enabled?"=TRUE, "Is.Connected?"=FALSE, "Device SN"="45876539", "AccelerationMaximum"=0.0, "VelocityMaximum"=0.0, "Acceleration"=0.0, "Velocity"=0.0, "waitTimeout (ms)"=0, "Model"=enum."Thorlabs MLJ", "Is.Homed?"=FALSE} ("Cluster In"), "Device SN"=w371) -> (w370:T2)
                                n123 = call "Thorlabs MLJ - Z Stage Module.vi"("Set/Get"=Set_Get_Controls."Set", "Error In"=w374, "Action"=w373, "Cluster In"=w370) -> ("Error Out"=w375:errorcluster)  [unwired: 6 in, 1 out]
                              }
                            }
                          }
                          frame 3 {
                            # "Vibratome Motor"
                          }
                        }
                      }
                      n124 = Merge Errors(w329) -> (w326:errorcluster)
                    }
                    frame Disabled {
                      w377 = Set_Get_Controls."Set" ("Set/Get")
                      w381 = Motion_Translation_Module_Control."Uninit" ("Action")
                      n125 = call "XYZ Table Stage Module.vi"("Set/Get"=w377, "Action"=w381, "Error In"=w389, "Axis"=enum16{"X Axis", "Y Axis", "Z Axis"}."X Axis") -> ("Error Out"=w388:errorcluster)  [unwired: 6 in, 1 out]
                      n126 = call "XYZ Table Stage Module.vi"("Set/Get"=w377, "Action"=w381, "Error In"=w388, "Axis"=enum16{"X Axis", "Y Axis", "Z Axis"}."Y Axis") -> ("Error Out"=w387:errorcluster)  [unwired: 6 in, 1 out]
                      n127 = call "XYZ Table Stage Module.vi"("Set/Get"=w377, "Action"=w381, "Error In"=w387, "Axis"=enum16{"X Axis", "Y Axis", "Z Axis"}."Z Axis") -> ("Error Out"=w384:errorcluster)  [unwired: 6 in, 1 out]
                      n128 = call "MCDC3006 Module.vi"("Actions"=T9."Disable Motor", "Error In"=w384) -> ("Error Out"=w383:errorcluster)  [unwired: 5 in, 4 out]
                      n129 = call "MCDC3006 Module.vi"("Actions"=T9."Close Session", "Error In"=w383) -> ("Error Out"=w382:errorcluster)  [unwired: 5 in, 4 out]
                    }
                  }
                }
                frame "Finished" {
                  n130 = Unbundle By Name(w394) -> ("Table Stages"=w395:T13)
                  n131 = Unbundle By Name(w394) -> ("Table Stages.X Stage.Velocity"=w396:dbl, "Vibratome.Slice Axis"=w393:enum16{"X Axis", "Y Axis", "Z Axis"})
                  n132 = case shown="\"Y Axis\"" w393 {
                    selector: w393 -> [w409 _ w418]
                    tunnel: w396 -> [w410 _ w419]
                    tunnel: w395 -> [w404 _ w413]
                    tunnel: [w408 w411 w417] -> w390
                    tunnel: w391 -> [w405 w411 w414]
                    frame "X Axis" {
                      n133 = Bundle By Name(cluster=w404, "X Stage.Velocity"=w410) -> (w403:T13)
                      n134 = call "XYZ Table Stage Module.vi"("Set/Get"=Set_Get_Controls."Set", "Action"=Motion_Translation_Module_Control."Velocity/Accel", "Error In"=w405, "Axis"=w409, "Table Stages"=w403) -> ("Error Out"=w408:errorcluster)  [unwired: 5 in, 1 out]
                    }
                    frame "Z Axis" {
                    }
                    frame "Y Axis" {
                      n135 = Bundle By Name(cluster=w413, "Y Stage.Velocity"=w419) -> (w412:T13)
                      n136 = call "XYZ Table Stage Module.vi"("Set/Get"=Set_Get_Controls."Set", "Action"=Motion_Translation_Module_Control."Velocity/Accel", "Error In"=w414, "Axis"=w418, "Table Stages"=w412) -> ("Error Out"=w417:errorcluster)  [unwired: 5 in, 1 out]
                    }
                  }
                  n137 = call "Inline Wait.vi"("Error In"=w390, "milliseconds to wait"=u32 10000) -> ("Error Out"=w399:errorcluster)  [unwired: 9 in]
                  n138 = call "FGV - Acquisition Status.vi"("Actions"=FGV_Actions."Set", "error in (no error)"=w399, "Action"=Thorlabs_Acq_Status."Idle") -> ("error out"=w398:errorcluster)  [unwired: 7 in, 1 out]
                }
              }
              n139 = case shown="Error" w20 {
                selector: w20 -> [w27 w28]
                tunnel: [w27 w28] -> w19
                tunnel: w18 -> [w26 w31]
                tunnel: [w25 w29] -> w17
                frame No Error {
                  n140 = Delete From Array(array=w26, index=0) -> (array with subset deleted=w25:string[])  [unwired: 1 in, 1 out]
                }
                frame Error {
                  n141 = Build Array (concatenate)("Error", w31) -> (w29:string[])
                }
              }
            }
          }
          frame Error {
          }
        }
        "error out" <- w5
      }
      frame "Image" {
        n142 = Wait (ms)(milliseconds to wait=u32 1000) -> ()  [unwired: 1 out]
      }
    }
  }
